vi "Sequence.GenerateSequence.vi"(8 "error in (no error)":errorcluster, 10 "Compiled Settings":T1, 11 "Path":path) -> (0 "error out":errorcluster)   [LabVIEW 2013, in "Simple Sequence Tools - Editor.lvlib"]
uses:
  Simple Sequence Tools - Editor.lvlib
  Types/Compiled.RTSequenceProperties.ctl
  Shared/Types/ChannelProperties.ctl
  Types/Compiled.StepProperties.ctl
  Types/Compiled.IOStateProperties.ctl
  Types/Compiled.StepElementProperties.ctl
  Shared/Types/StepTypes.ctl
  Types/Compiled.StepCondition.ctl
  Types/OperationTypes.ctl
  Types/Compiled.SequenceChannels.ctl
  NationalInstruments.VeriStand.RealTimeSequenceDefinitionApi
  Shared/Simple Sequence Tools - Shared.lvlib
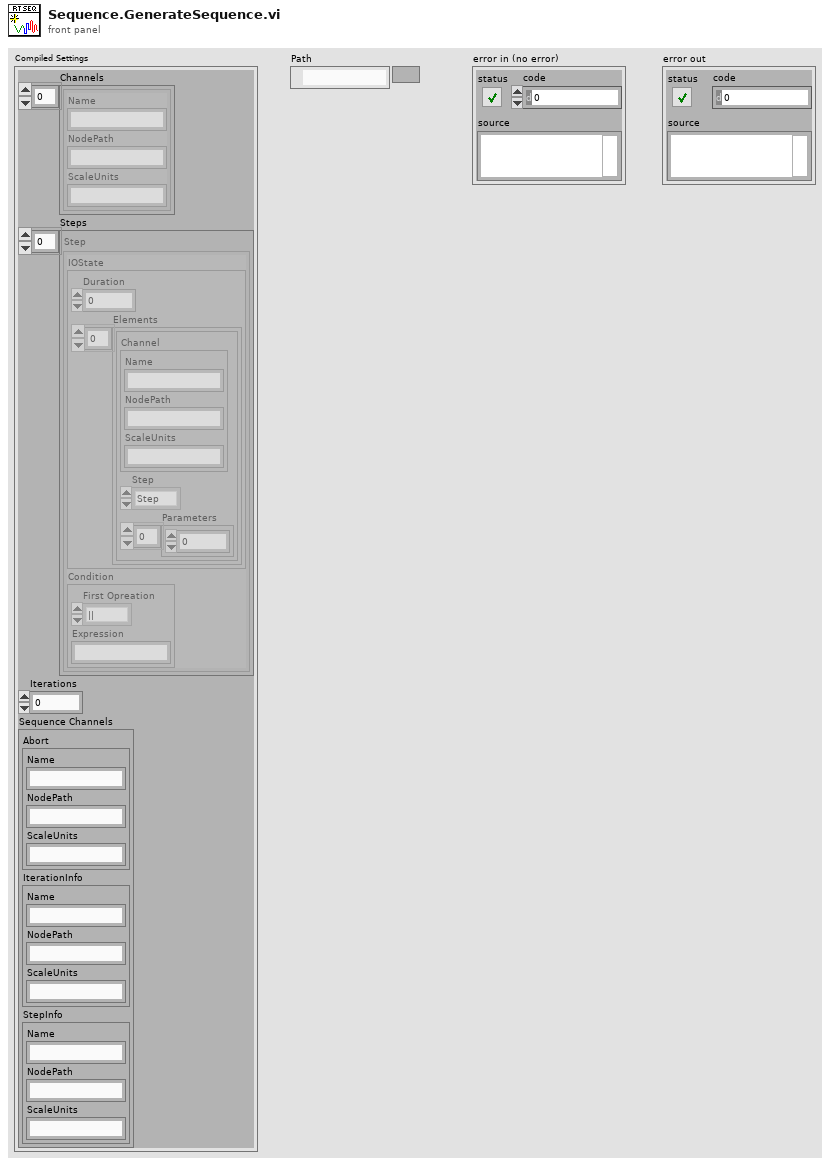
[diagram p1: front panel]
types:
  T1 = typedef "Simple Sequence Tools - Editor.lvlib/Compiled.RTSequenceProperties.ctl" = cluster{"Channels":T2[], "Steps":T3[], "Iterations":u32, "Sequence Channels":T9}
  T2 = typedef "Simple Sequence Tools - Shared.lvlib/ChannelProperties.ctl" = cluster{"Name":string, "NodePath":string, "ScaleUnits":string}
  T3 = typedef "Simple Sequence Tools - Editor.lvlib/Compiled.StepProperties.ctl" = cluster{"IOState":T4, "Condition":T7}
  T4 = typedef "Simple Sequence Tools - Editor.lvlib/Compiled.IOStateProperties.ctl" = cluster{"Duration":dbl, "Elements":T5[]}
  T5 = typedef "Simple Sequence Tools - Editor.lvlib/Compiled.StepElementProperties.ctl" = cluster{"Channel":T2, "Step":T6, "Parameters":dbl[]}
  T6 = typedef "Simple Sequence Tools - Shared.lvlib/StepTypes.ctl" = enum8{"Step", "iStep", "Ramp", "Unchanged", "Unknown"}
  T7 = typedef "Simple Sequence Tools - Editor.lvlib/Compiled.StepCondition.ctl" = cluster{"First Opreation":T8, "Expression":string}
  T8 = typedef "Simple Sequence Tools - Editor.lvlib/OperationTypes.ctl" = enum8{"None", "&&", "||"}
  T9 = typedef "Simple Sequence Tools - Editor.lvlib/Compiled.SequenceChannels.ctl" = cluster{"Abort":T2, "IterationInfo":T2, "StepInfo":T2}
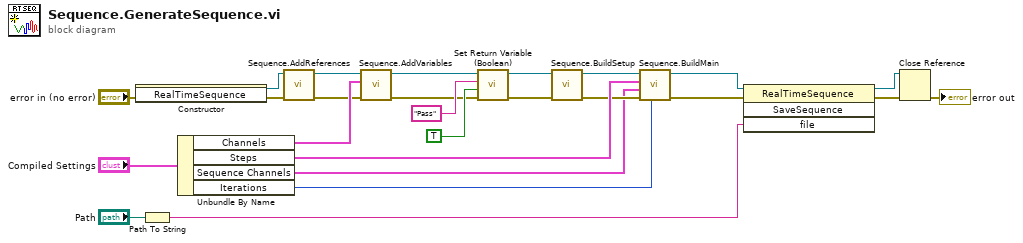
[diagram p0: block diagram]
diagram:
  n1 = constructor class="RealTimeSequence"(error in="error in (no error)") -> (reference out=w13:refnum<k24>, error out=w3:errorcluster)  [unwired: 2 in, 1 out]
  n2 = Path To String(path="Path") -> (string=w15:string)
  n3 = Unbundle By Name("Compiled Settings") -> ("Channels"=w21:T2[], "Steps"=w10:T3[], "Sequence Channels"=w2:T9, "Iterations"=w1:u32)
  n4 = call "Sequence.AddReferences.vi"("error in (no error)"=w3, "Sequence"=w13) -> ("error out"=w11:errorcluster, "Sequence out"=w12:refnum<k24>)  [unwired: 8 in]
  n5 = call "Sequence.AddVariables.vi"("error in (no error)"=w11, "Channels"=w21, "Sequence"=w12) -> ("error out"=w20:errorcluster, "Sequence out"=w19:refnum<k24>)  [unwired: 7 in]
  n6 = call "Set Return Variable (Boolean).vi"("error in (no error)"=w20, "Value"=TRUE, "Identifier"="Pass", "Sequence Ref in"=w19) -> ("error out"=w8:errorcluster, "Sequence Ref out"=w7:refnum<k24>)  [unwired: 6 in]
  n7 = call "Sequence.BuildSetup.vi"("error in (no error)"=w8, "Sequence"=w7) -> ("error out"=w5:errorcluster, "Sequence out"=w6:refnum<k24>)  [unwired: 8 in]
  n8 = call "Sequence.BuildMain.vi"("Iterations"=w1, "error in (no error)"=w5, "Sequence Channels"=w2, "Steps"=w10, "Sequence"=w6) -> ("error out"=w9:errorcluster, "Sequence out"=w14:refnum<k24>)  [unwired: 5 in]
  n9 = invoke class="RealTimeSequence" method="SaveSequence"(reference=w14, error in=w9, "file"=w15) -> (reference out=w25:refnum<k24>, error out=w18:errorcluster)  [unwired: 1 in, 2 out]
  n10 = Close Reference(reference=w25, error in (no error)=w18) -> (error out=→"error out":errorcluster)
